vi "Tool Simulator Q.vi"(11 "error in (no error)":errorcluster) -> (6 "Tool data Q":refnum<queue>, 8 "Tool Data not":refnum<notifier>, 15 "error out":errorcluster)   [LabVIEW 2011]
uses:
  Tool simulator data.ctl
  Measurments Handling/Status Digitalish.ctl
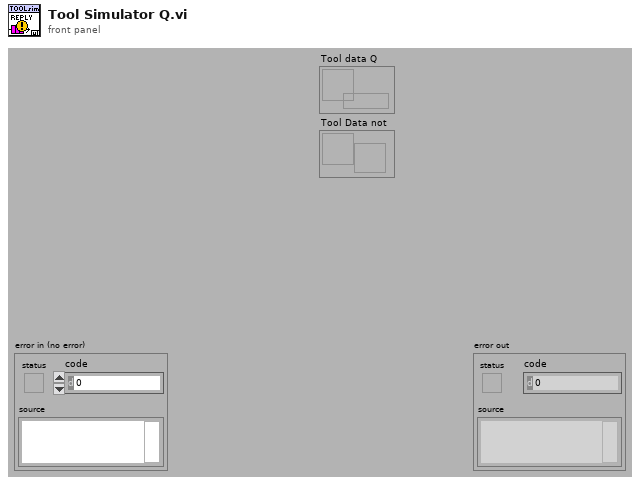
[diagram p1: front panel]
types:
  T1 = typedef "Tool simulator data.ctl" = cluster{"Analog Values":dbl[], "Digital Values":T2[]}
  T2 = typedef "Status Digitalish.ctl" = enum16{"NA", "False", "True"}
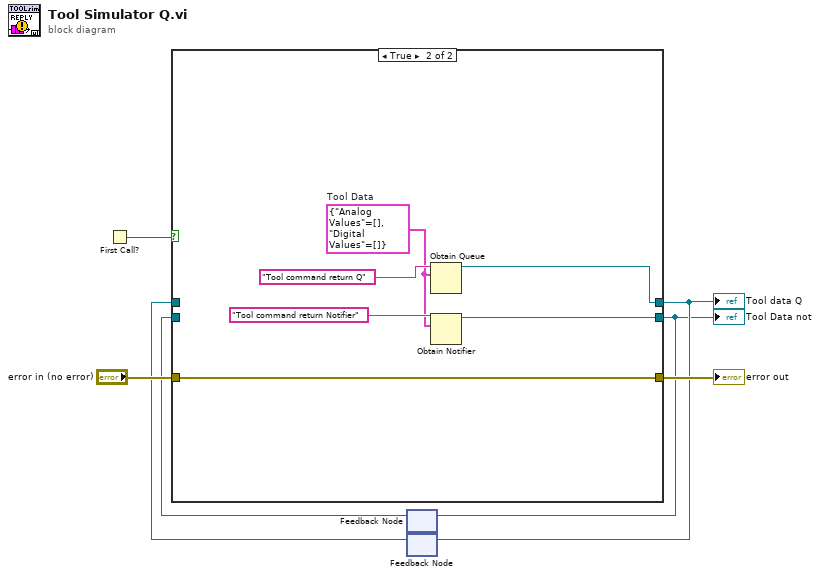
[diagram p0: block diagram]
diagram:
  n1 = First Call?() -> (First Call?: T/F=w5:bool)
  n2 = feedback #1() -> (w2:refnum<notifier>)  [unwired: 1 in]
  n3 = feedback #2() -> (w3:refnum<queue>)  [unwired: 1 in]
  n4 = case shown="True" w5 {
    tunnel: [w10 w16] -> w7
    tunnel: "error in (no error)" -> [w10 w16]
    tunnel: [w9 w14] -> w4
    tunnel: w3 -> [w9 _]
    tunnel: [w8 w12] -> w1
    tunnel: w2 -> [w8 _]
    frame False {
    }
    frame True {
      w11 = T1 {"Analog Values"=[], "Digital Values"=[]}  # Tool Data
      n5 = Obtain Queue(name (unnamed)="Tool command return Q", element data type=w11) -> (queue out=w14:refnum<queue>)  [unwired: 3 in, 2 out]
      n6 = Obtain Notifier(name (unnamed)="Tool command return Notifier", notification data type=w11) -> (notifier out=w12:refnum<notifier>)  [unwired: 2 in, 2 out]
    }
  }
  "error out" <- w7
  "Tool data Q" <- w4
  "Tool Data not" <- w1
  n7 = feedback-in #1(w1) -> ()
  n8 = feedback-in #2(w4) -> ()
